vi "无人机外部环境监测.vi"() -> ()   [LabVIEW 2024]
uses:
  <vilib>/Utility/file.llb/Read Delimited Spreadsheet (DBL).vi
panel:
  out "湿度":dbl(knob) scale=0.0..100.0
  out "温度":dbl(knob) scale=0.0..100.0
  out "Z数组":dbl[](array[numeric])
  out "Y数组":dbl[](array[numeric])
  out "X数组":dbl[](array[numeric])
  in  "停止":bool
  in  "开始":bool
  out "报警灯":bool
  in  "加速度":path
  out "当前加速度":dbl
  out "报警灯":bool
  in  "湿度":path
  out "报警灯":bool
  in  "温度":path
  in  "加速度上限":dbl
  in  "加速度下限":dbl
  in  "湿度上限":dbl
  in  "湿度下限":dbl
  in  "温度上限":dbl
  in  "温度下限":dbl
  out "加速度":cluster{"加速度上限":dbl, dbl, dbl, dbl, "加速度下限":dbl}(graph)
  out "湿度":cluster{dbl, "温度上限":dbl, "温度下限":dbl}(graph)
  out "温度":cluster{dbl, "温度上限":dbl, "温度下限":dbl}(graph)
  # "无人机外部环境检测系统"
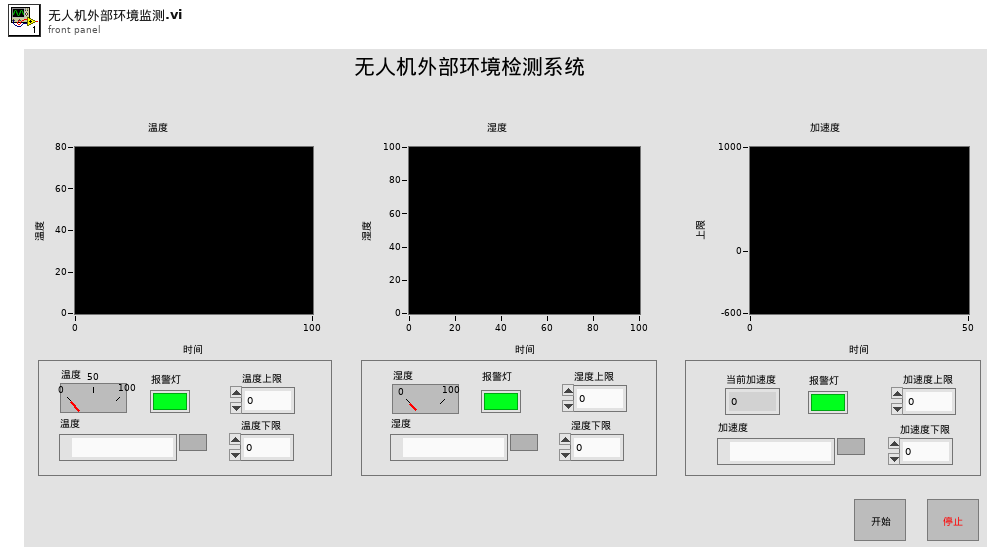
[diagram p1: front panel]
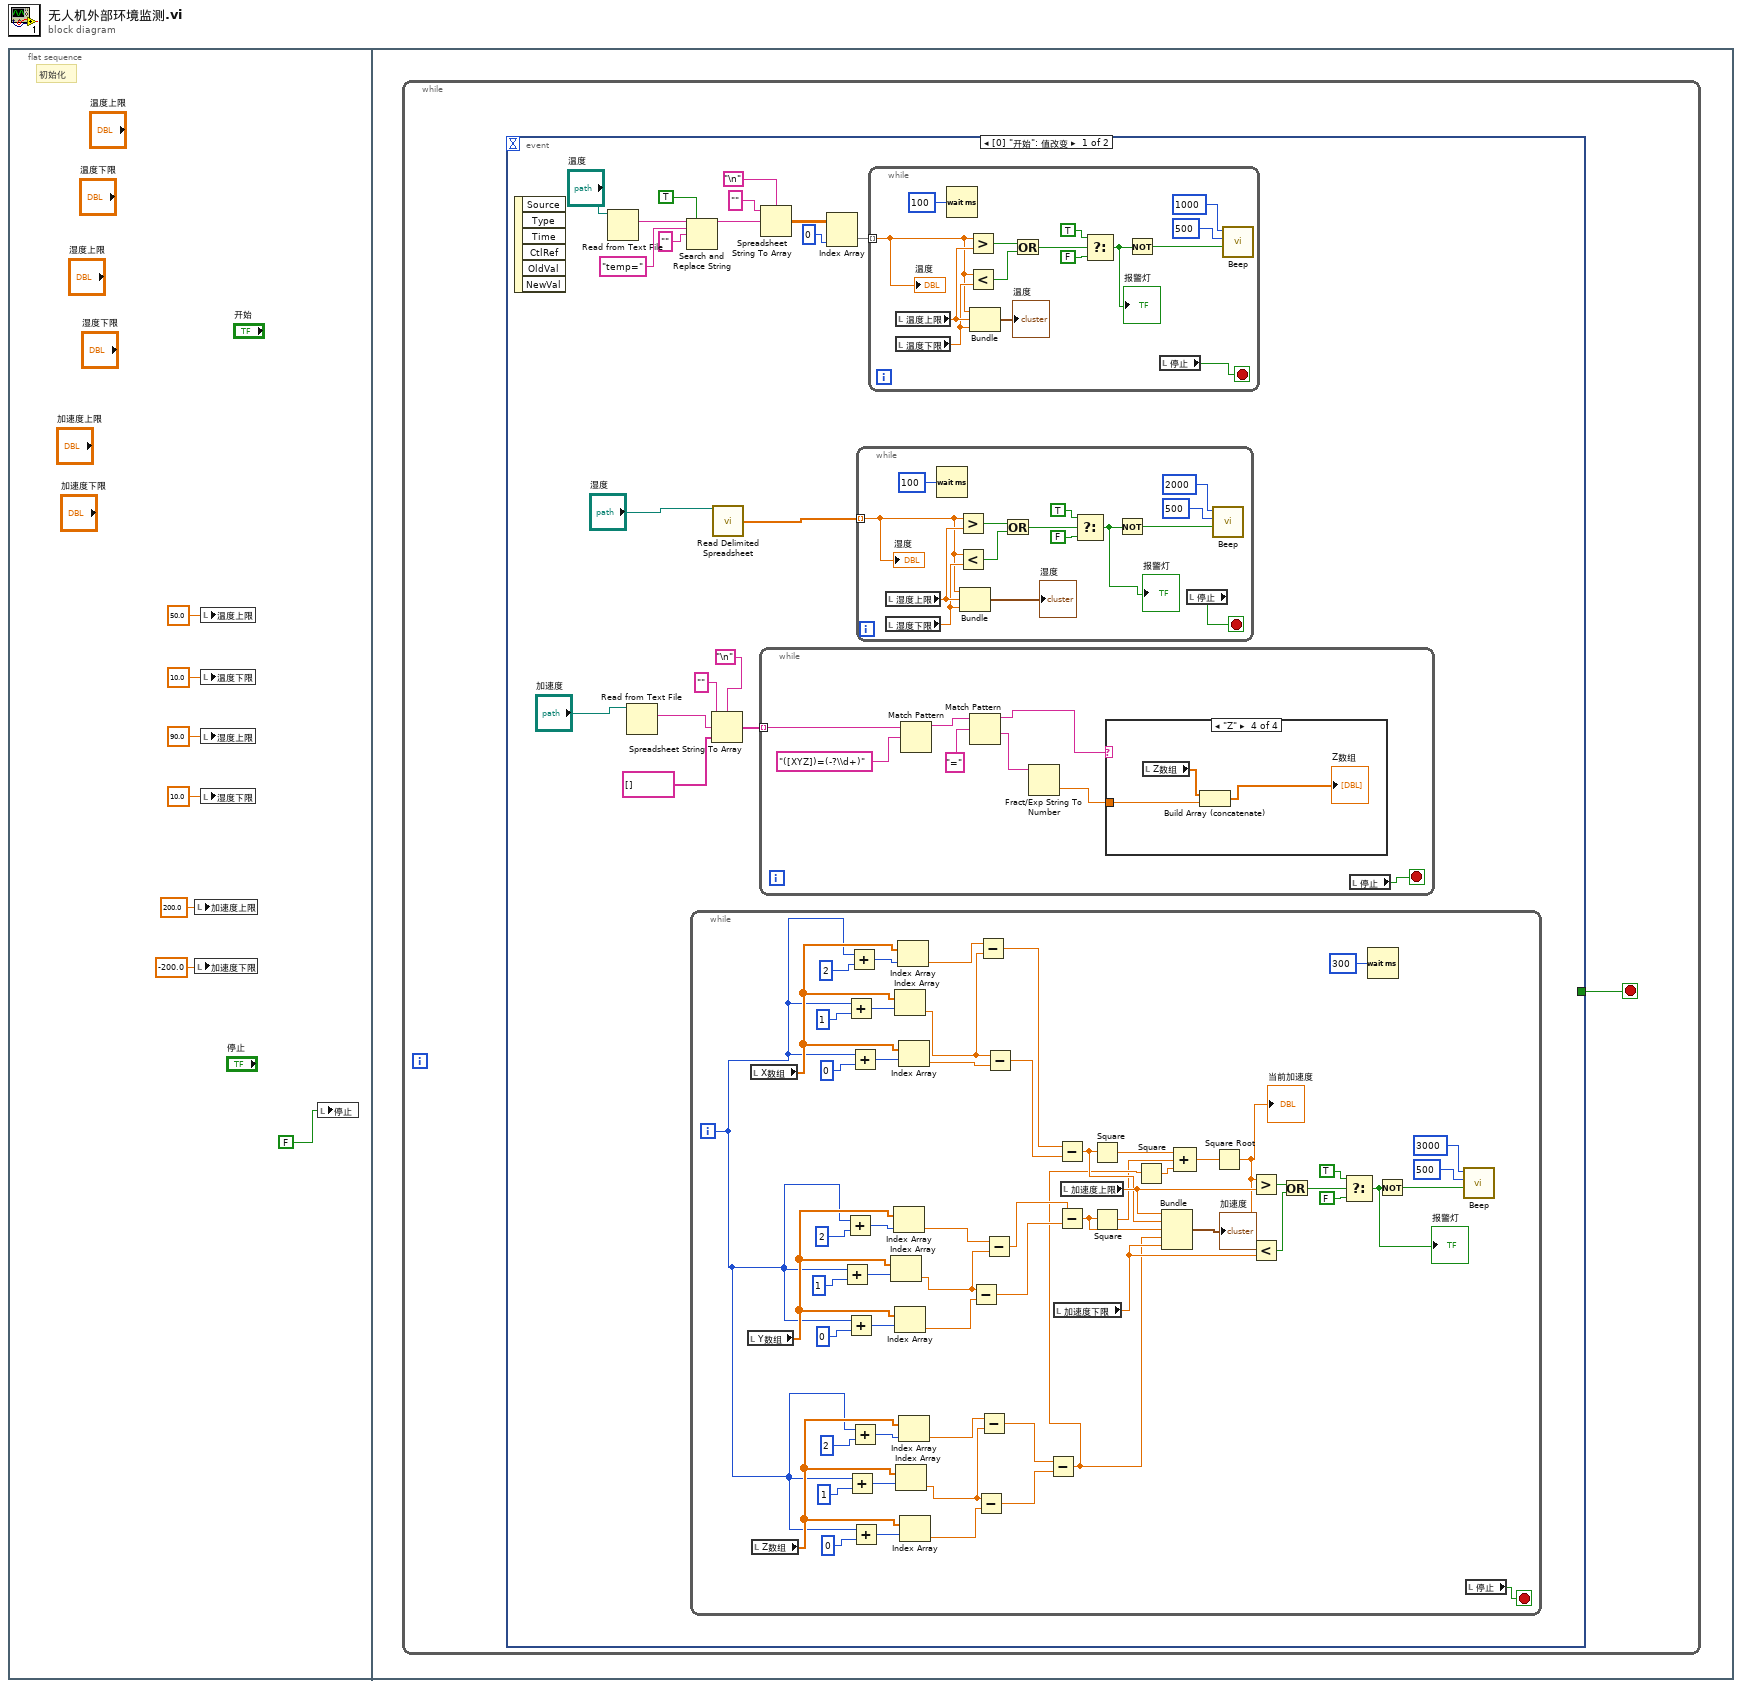
[diagram p0: block diagram]
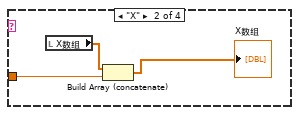
[diagram p3: hidden frame]
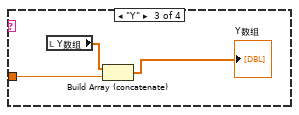
[diagram p4: hidden frame]
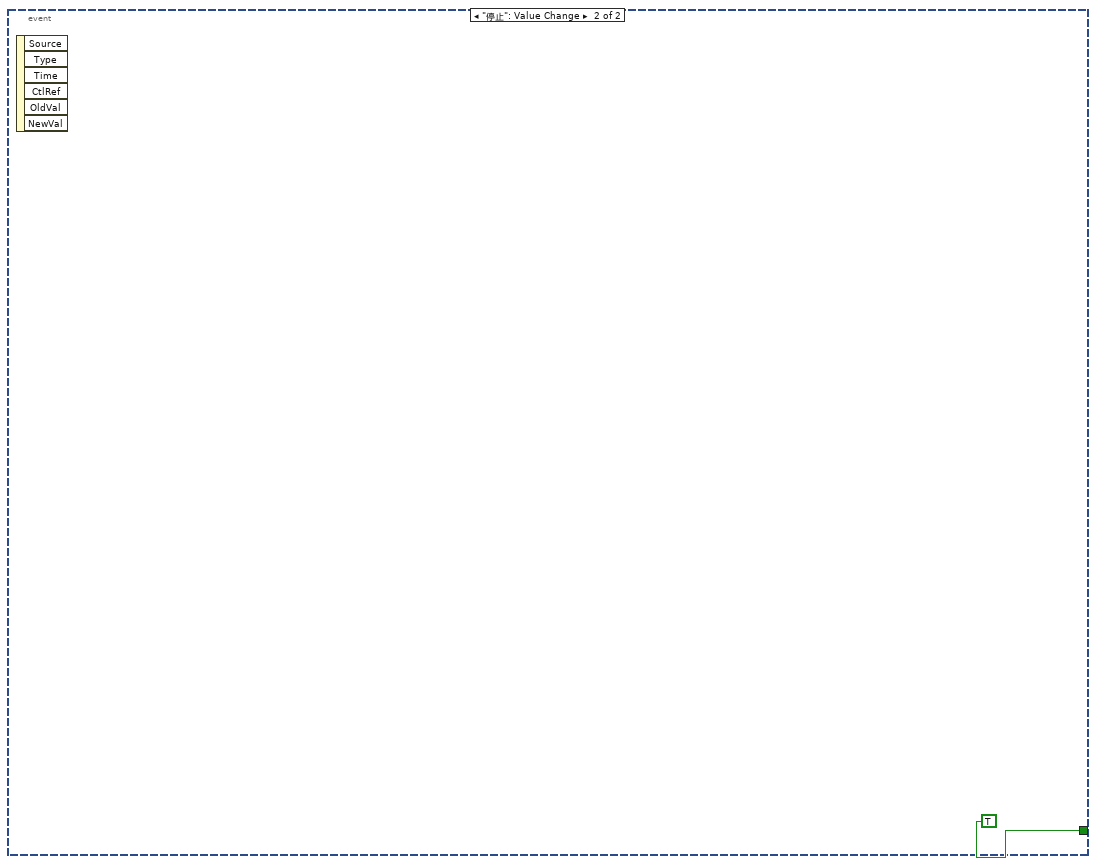
[diagram p5: hidden frame]
diagram:
  n1 = flat-sequence {
    frame #0 {
      # "初始化"
      n2 = local write "加速度上限"(200.0 ("温度上限")) -> ()
      n3 = local write "加速度下限"(-200.0 ("温度下限")) -> ()
      n4 = local write "温度上限"(50.0 ("温度上限")) -> ()
      n5 = local write "温度下限"(10.0 ("温度下限")) -> ()
      n6 = local write "湿度上限"(90.0 ("温度上限")) -> ()
      n7 = local write "湿度下限"(10.0 ("温度下限")) -> ()
      n8 = local write "停止"(FALSE ("停止")) -> ()
    }
    frame #1 {
      n9 = while {
        stop <- w8 stop-if-true
        n10 = event shown="[0] \"开始\": 值改变" {
          selector: _ -> [_ _]
          dyn-events: _ -> [_ _]
          timeout: _ -> [_ _]
          tunnel: [_ TRUE ("停止")] -> w8
          event "开始": Value Change {
            n11 = event-data() -> ()  [unwired: 1 in, 6 out]
            n12 = Read from Text File(file (use dialog)="温度") -> (text=w24:string)  [unwired: 3 in, 3 out]
            n13 = Read from Text File(file (use dialog)="加速度") -> (text=w13:string)  [unwired: 3 in, 3 out]
            n14 = Search and Replace String(replace all?=TRUE ("替换全部？(F)"), input string=w24, search string="temp=" ("搜索字符串"), replace string="" ("替换字符串(\"\")")) -> (result string=w20:string)  [unwired: 4 in, 3 out]
            n15 = while {
              i -> [w95]
              stop <- w75 stop-if-true
              n16 = local read "Y数组"() -> (w114:dbl[])
              n17 = local read "X数组"() -> (w127:dbl[])
              n18 = local read "Z数组"() -> (w101:dbl[])
              n19 = Add(x=w95, y=1) -> (x+y=w111:i32)
              n20 = Add(x=w95, y=2) -> (x+y=w108:i32)
              n21 = Add(x=w95, y=1) -> (x+y=w130:i32)
              n22 = Add(x=w95, y=0) -> (x+y=w113:i32)
              n23 = Add(x=w95, y=1) -> (x+y=w104:i32)
              n24 = Add(x=w95, y=2) -> (x+y=w133:i32)
              n25 = Add(x=w95, y=0) -> (x+y=w128:i32)
              n26 = Add(x=w95, y=2) -> (x+y=w107:i32)
              n27 = Add(x=w95, y=0) -> (x+y=w102:i32)
              n28 = Index Array(array=w114, index=w111) -> (element=w117:dbl)
              n29 = Index Array(array=w114, index=w108) -> (element=w116:dbl)
              n30 = Index Array(array=w127, index=w130) -> (element=w124:dbl)
              n31 = Index Array(array=w114, index=w113) -> (element=w115:dbl)
              n32 = Index Array(array=w101, index=w104) -> (element=w98:dbl)
              n33 = Index Array(array=w127, index=w133) -> (element=w125:dbl)
              n34 = Index Array(array=w127, index=w128) -> (element=w126:dbl)
              n35 = Index Array(array=w101, index=w107) -> (element=w99:dbl)
              n36 = Index Array(array=w101, index=w102) -> (element=w100:dbl)
              n37 = Subtract(x=w117, y=w115) -> (x-y=w119:dbl)
              n38 = Subtract(x=w98, y=w100) -> (x-y=w96:dbl)
              n39 = Subtract(x=w125, y=w124) -> (x-y=w122:dbl)
              n40 = Subtract(x=w99, y=w98) -> (x-y=w97:dbl)
              n41 = Subtract(x=w116, y=w117) -> (x-y=w118:dbl)
              n42 = Subtract(x=w124, y=w126) -> (x-y=w121:dbl)
              n43 = Subtract(x=w97, y=w96) -> (x-y=w81:dbl)
              n44 = local read "加速度下限"() -> (w85:dbl)
              n45 = Subtract(x=w122, y=w121) -> (x-y=w84:dbl)
              n46 = Subtract(x=w118, y=w119) -> (x-y=w82:dbl)
              n47 = local read "加速度上限"() -> (w86:dbl)
              n48 = Square(x=w84) -> (x^2=w83:dbl)
              n49 = Square(x=w82) -> (x^2=w80:dbl)
              n50 = Square(x=w81) -> (x^2=w79:dbl)
              n51 = Bundle("加速度上限"=w86, w84, w82, w81, "加速度下限"=w85) -> (→"加速度":cluster{"加速度上限":dbl, dbl, dbl, dbl, "加速度下限":dbl})  [unwired: 1 in]
              n52 = Compound Arithmetic op=ADD(w83, w80, w79) -> (w78:dbl)
              n53 = Square Root(x=w78) -> (sqrt(x)=w76:dbl)
              "当前加速度" <- w76
              n54 = Greater?(x=w76, y=w86) -> (0:w89:bool)
              n55 = Less?(x=w76, y=w85) -> (x < y?=w87:bool)
              n56 = Or(x=w89, y=w87) -> (x .or. y?=w90:bool)
              n57 = Select(t=TRUE, s=w90, f=FALSE) -> (s? t:f=w77:bool)
              "报警灯" <- w77
              n58 = Wait (ms)(milliseconds to wait=u32 300 ("等待时间（毫秒）")) -> ()  [unwired: 1 out]
              n59 = Not(x=w77) -> (.not. x?=w94:bool)
              n60 = call <vilib>:"Beep.vi"("use system alert? (T)"=w94, "duration (msec)"=u32 500, "frequency (Hz)"=u32 3000) -> ()  [unwired: 9 in]
              n61 = local read "停止"() -> (w75:bool)
            }
            n62 = Spreadsheet String To Array(delimiter (Tab)="\n", format string="" ("格式字符串"), spreadsheet string=w13, array type (2D Dbl)=string[] []) -> (array=w9:string[])
            n63 = call-poly <vilib>:"Read Delimited Spreadsheet.vi"("file path (dialog if empty)"="湿度") -> ("first row"=w14:dbl[])  [unwired: 9 in, 5 out]
            n64 = while {
              tunnel: w9 -> [w65] mode=indexing
              stop <- w58 stop-if-true
              n65 = Match Pattern(string=w65, regular expression="([XYZ])=(-?\\d+)" ("正则表达式")) -> (before substring=w59:string)  [unwired: 1 in, 3 out]
              n66 = Match Pattern(string=w59, regular expression="=" ("正则表达式")) -> (before substring=w60:string, after substring=w61:string)  [unwired: 1 in, 2 out]
              n67 = Fract/Exp String To Number(string=w61) -> (number=w62:dbl)  [unwired: 3 in, 1 out]
              n68 = case shown="\"Z\"" w60 {
                tunnel: w62 -> [_ w66 w69 w72]
                frame "0", Default {
                }
                frame "X" {
                  n69 = local read "X数组"() -> (w68:dbl[])
                  n70 = Build Array (concatenate)(w68, w66) -> (→"X数组":dbl[])
                }
                frame "Y" {
                  n71 = local read "Y数组"() -> (w71:dbl[])
                  n72 = Build Array (concatenate)(w71, w69) -> (→"Y数组":dbl[])
                }
                frame "Z" {
                  n73 = local read "Z数组"() -> (w74:dbl[])
                  n74 = Build Array (concatenate)(w74, w72) -> (→"Z数组":dbl[])
                }
              }
              n75 = local read "停止"() -> (w58:bool)
            }
            n76 = Spreadsheet String To Array(delimiter (Tab)="\n", format string="" ("格式字符串"), spreadsheet string=w20) -> (array=w18:dbl[][])  [unwired: 1 in]
            n77 = Index Array(array=w18, index (col)=0 ("索引 (列)")) -> (element=w27:dbl[])  [unwired: 1 in]
            n78 = while {
              tunnel: w14 -> [w43] mode=indexing
              stop <- w44 stop-if-true
              n79 = local read "湿度上限"() -> (w51:dbl)
              n80 = local read "湿度下限"() -> (w50:dbl)
              n81 = Wait (ms)(milliseconds to wait=u32 100 ("等待时间（毫秒）")) -> ()  [unwired: 1 out]
              n82 = Greater?(x=w43, y=w51) -> (0:w56:bool)
              n83 = Less?(x=w43, y=w50) -> (x < y?=w57:bool)
              n84 = Bundle("Numeric"=w43, "湿度上限"=w51, "湿度下限"=w50) -> (→"湿度":cluster{"Numeric":dbl, "湿度上限":dbl, "湿度下限":dbl})  [unwired: 1 in]
              n85 = Or(x=w56, y=w57) -> (x .or. y?=w55:bool)
              n86 = Select(t=TRUE, s=w55, f=FALSE) -> (s? t:f=w45:bool)
              "报警灯" <- w45
              n87 = Not(x=w45) -> (.not. x?=w47:bool)
              n88 = local read "停止"() -> (w44:bool)
              n89 = call <vilib>:"Beep.vi"("use system alert? (T)"=w47, "duration (msec)"=u32 500, "frequency (Hz)"=u32 2000) -> ()  [unwired: 9 in]
              "湿度" <- w43
            }
            n90 = while {
              tunnel: w27 -> [w28] mode=indexing
              stop <- w29 stop-if-true
              n91 = local read "温度上限"() -> (w35:dbl)
              n92 = local read "温度下限"() -> (w34:dbl)
              n93 = Wait (ms)(milliseconds to wait=u32 100 ("等待时间（毫秒）")) -> ()  [unwired: 1 out]
              n94 = Greater?(x=w28, y=w35) -> (0:w41:bool)
              n95 = Less?(x=w28, y=w34) -> (x < y?=w42:bool)
              n96 = Bundle(w28, "温度上限"=w35, "温度下限"=w34) -> (→"温度":cluster{dbl, "温度上限":dbl, "温度下限":dbl})  [unwired: 1 in]
              n97 = Or(x=w41, y=w42) -> (x .or. y?=w40:bool)
              n98 = Select(t=TRUE, s=w40, f=FALSE) -> (s? t:f=w30:bool)
              "报警灯" <- w30
              n99 = Not(x=w30) -> (.not. x?=w31:bool)
              n100 = local read "停止"() -> (w29:bool)
              n101 = call <vilib>:"Beep.vi"("use system alert? (T)"=w31, "duration (msec)"=u32 500, "frequency (Hz)"=u32 1000) -> ()  [unwired: 9 in]
              "温度" <- w28
            }
          }
          event "停止": Value Change {
            n102 = event-data() -> ()  [unwired: 1 in, 6 out]
          }
        }
      }
    }
  }
